vi "CreateModuleEvents.vi"(8 "error in (no error)":errorcluster) -> (0 "error out":errorcluster, 3 "Broadcasts":T1)   [LabVIEW 2024, in "TesterModule.lvclass"]
uses:
  TesterModule.lvclass/TesterModule.ctl
  TesterModule.lvclass
  Stopped.ctl
  Broadcasts.ctl
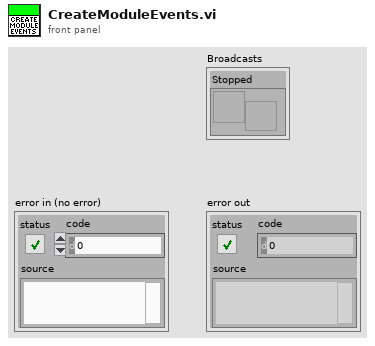
[diagram p1: front panel]
types:
  T1 = typedef "TesterModule.lvclass/Broadcasts.ctl" = cluster{"Stopped":refnum<user-event>}
  T2 = typedef "TesterModule.lvclass/Stopped.ctl" = bool
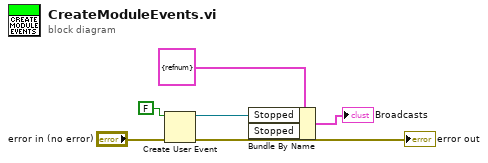
[diagram p0: block diagram]
diagram:
  n1 = Create User Event(user event datatype=T2 FALSE ("Stopped"), error in="error in (no error)") -> (user event=w4:refnum<user-event>, error out=→"error out":errorcluster)
  n2 = Bundle By Name(cluster=T1 {"Stopped"=refnum} ("Broadcasts"), "Stopped"=w4) -> (→"Broadcasts":T1)  [unwired: 1 in]
